vi "Write File Setup.vi"(8 "error in (no error)":errorcluster, 10 "Setup":T1, 11 "Setup File in":refnum<class "Setup File.lvclass">) -> (0 "error out":errorcluster, 3 "Setup File out":refnum<class "Setup File.lvclass">)   [LabVIEW 2018, in "Setup File.lvclass"]
uses:
  Setup File.lvclass
  Setup File.lvclass/Setup File.ctl
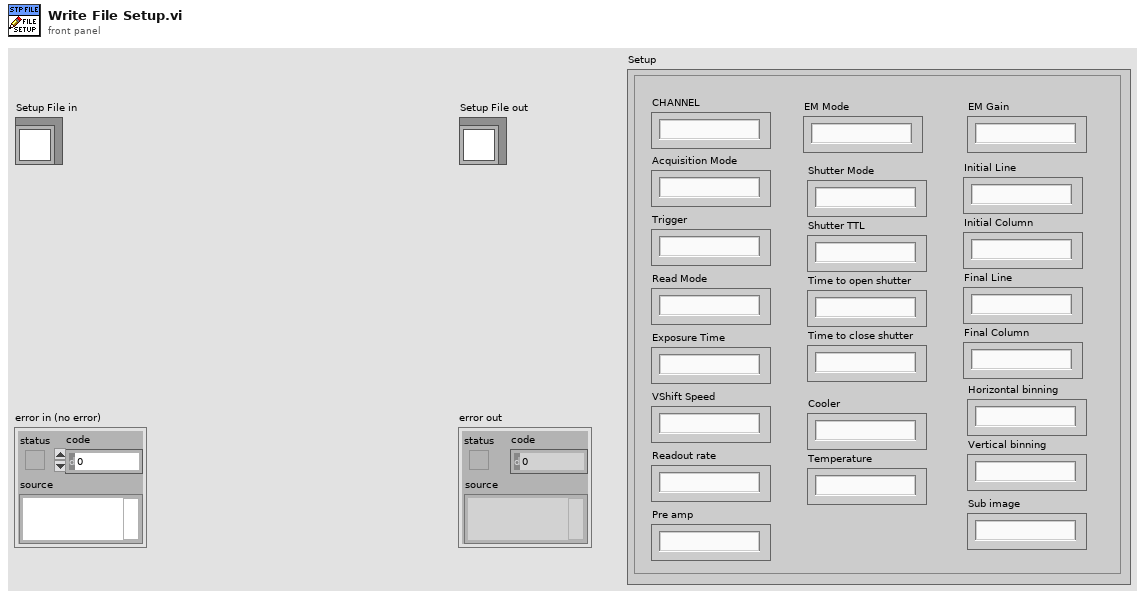
[diagram p1: front panel]
types:
  T1 = cluster{"Read Mode":string, "Acquisition Mode":string, "Trigger":string, "Exposure Time":string, "VShift Speed":string, "Readout rate":string, "Pre amp":string, "Shutter Mode":string, "Shutter TTL":string, "Time to open shutter":string, "Time to close shutter":string, "Cooler":string, "Temperature":string, "Initial Line":string, "Initial Column":string, "Final Line":string, "Final Column":string, "Horizontal binning":string, "Vertical binning":string, "Sub image":string, "CHANNEL":string, "EM Mode":string, "EM Gain":string}
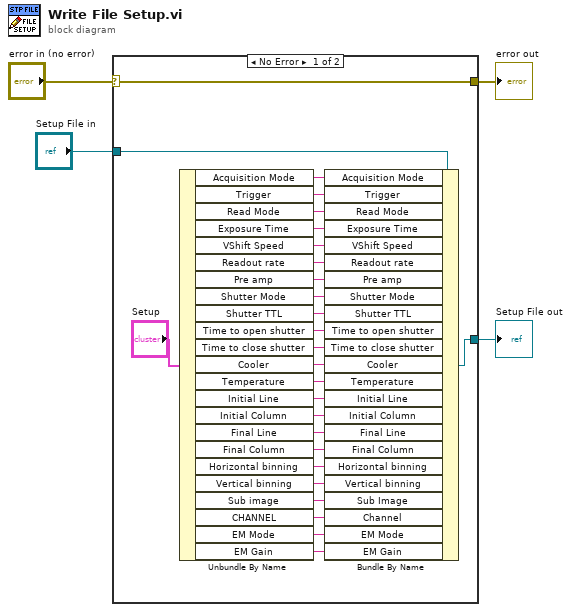
[diagram p0: block diagram]
diagram:
  n1 = case shown="No Error" "error in (no error)" {
    selector: "error in (no error)" -> [w31 w32]
    tunnel: [w31 w32] -> w2
    tunnel: [w29 w33] -> w3
    tunnel: "Setup File in" -> [w30 w33]
    frame No Error {
      n2 = Unbundle By Name("Setup") -> ("Acquisition Mode"=w9:string, "Trigger"=w10:string, "Read Mode"=w11:string, "Exposure Time"=w12:string, "VShift Speed"=w13:string, "Readout rate"=w14:string, "Pre amp"=w15:string, "Shutter Mode"=w16:string, "Shutter TTL"=w17:string, "Time to open shutter"=w18:string, "Time to close shutter"=w19:string, "Cooler"=w20:string, "Temperature"=w21:string, "Initial Line"=w22:string, "Initial Column"=w23:string, "Final Line"=w24:string, "Final Column"=w25:string, "Horizontal binning"=w26:string, "Vertical binning"=w27:string, "Sub image"=w8:string, "CHANNEL"=w7:string, "EM Mode"=w5:string, "EM Gain"=w6:string)
      n3 = Bundle By Name(cluster=w30, "Acquisition Mode"=w9, "Trigger"=w10, "Read Mode"=w11, "Exposure Time"=w12, "VShift Speed"=w13, "Readout rate"=w14, "Pre amp"=w15, "Shutter Mode"=w16, "Shutter TTL"=w17, "Time to open shutter"=w18, "Time to close shutter"=w19, "Cooler"=w20, "Temperature"=w21, "Initial Line"=w22, "Initial Column"=w23, "Final Line"=w24, "Final Column"=w25, "Horizontal binning"=w26, "Vertical binning"=w27, "Sub Image"=w8, "Channel"=w7, "EM Mode"=w5, "EM Gain"=w6) -> (w29:refnum<class "Setup File.lvclass">)
    }
    frame Error {
    }
  }
  "error out" <- w2
  "Setup File out" <- w3
